vi "Append Waveforms.vi"(8 "Error In":errorcluster, 9 "Signals In":waveform(dbl)[](array[waveform])) -> (0 "Error Out":errorcluster, 1 "Appended Signals Out":waveform(dbl)[](array[waveform]))   [LabVIEW 2016]
panel:
  # "Append latest aqcuried signal block to the previous block.\nCreates a 50% overlap between successive acquisition blocks, \ne.g for improved spectrum calculations"
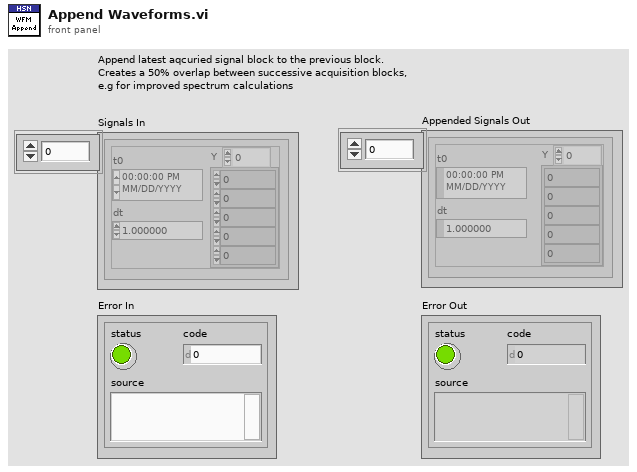
[diagram p1: front panel]
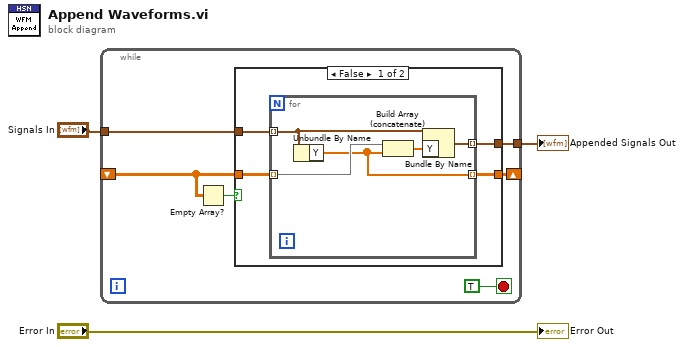
[diagram p0: block diagram]
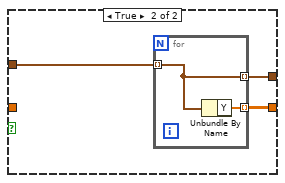
[diagram p2: hidden frame]
diagram:
  n1 = while {
    shift-right: [w9] -> _
    shift-left: _ -> [w4]
    tunnel: [w8] -> w2
    tunnel: "Signals In" -> [w6]
    stop <- TRUE stop-if-true
    n2 = Empty Array?(array=w4) -> (empty?=w5:bool)
    n3 = case shown="False" w5 {
      tunnel: [w13 w19] -> w9
      tunnel: [w12 w20] -> w8
      tunnel: w6 -> [w11 w21]
      tunnel: w4 -> [w10 _]
      frame False {
        n4 = for {
          tunnel: w11 -> [w16] mode=indexing
          tunnel: [w17] -> w13 mode=indexing
          tunnel: w10 -> [w18] mode=indexing
          tunnel: [w14] -> w12 mode=indexing
          n5 = Unbundle By Name(w16) -> ("Y"=w17:dbl[])
          n6 = Build Array (concatenate)(w18, w17) -> (w15:dbl[])
          n7 = Bundle By Name(cluster=w16, "Y"=w15) -> (w14:waveform(dbl))
        }
      }
      frame True {
        n8 = for {
          tunnel: w21 -> [w22] mode=indexing
          tunnel: [w23] -> w19 mode=indexing
          tunnel: [w22] -> w20 mode=indexing
          n9 = Unbundle By Name(w22) -> ("Y"=w23:dbl[])
        }
      }
    }
  }
  "Appended Signals Out" <- w2
  "Error Out" <- "Error In"
